vi "xml_lib Implementation.vi"(8 "error in (no error)":errorcluster, 11 "class path":path) -> (0 "error out":errorcluster, 3 "Array":path[](array[path]))   [LabVIEW 2020, in "Test Method Finding Test.lvclass"]
uses:
  Test Method Finding Test.lvclass
  <vilib>/xml/Load XML File.vi
  <vilib>/xml/Close Reference(Node).vi
  Test Method Finding Test.lvclass/Test Method Finding Test.ctl
  <resource>/objmgr/DOMUserDefRef.rc
  <vilib>/xml/NI_XML.lvlib
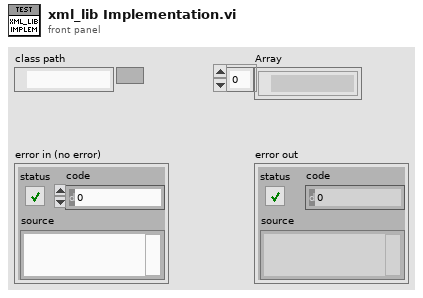
[diagram p1: front panel]
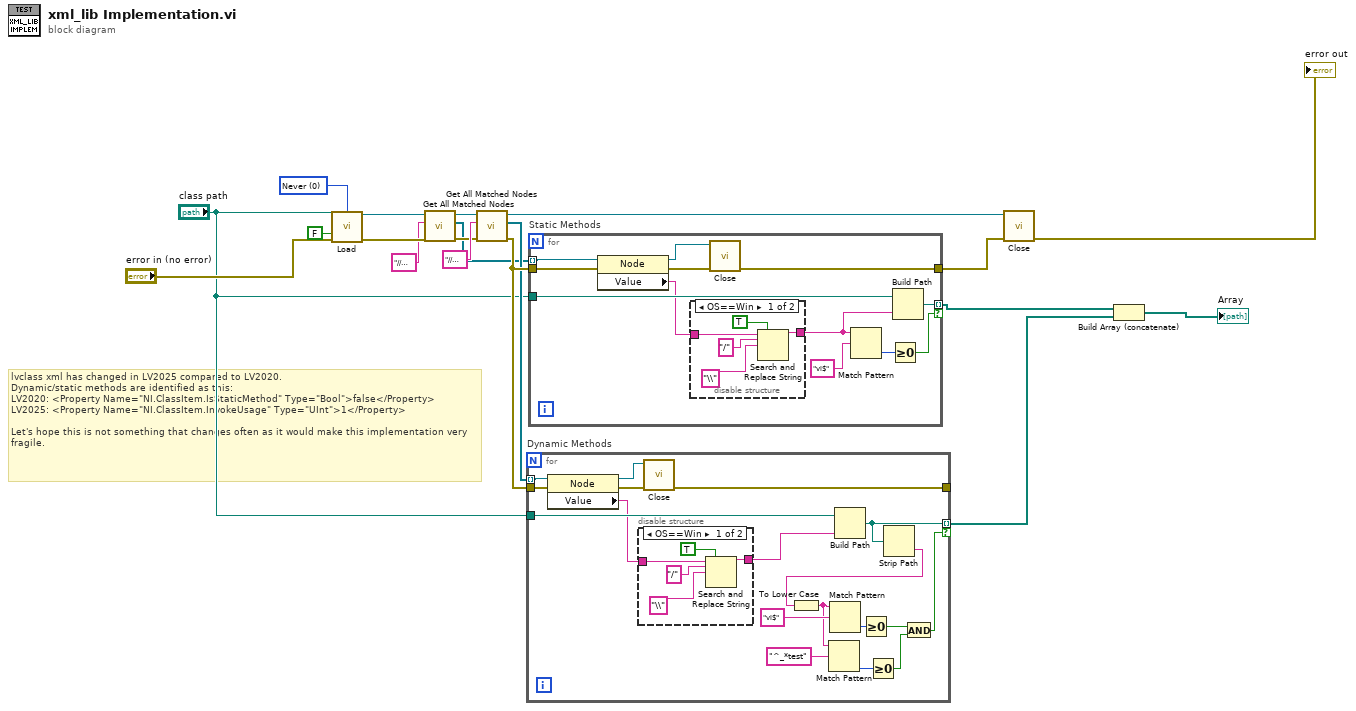
[diagram p0: block diagram]
diagram:
  w5 = 0 items=["Never", "Always", "Auto"] ("validate on load (Auto)")
  # "lvclass xml has changed in LV2025 compared to LV2020.\nDynamic/static methods are identified as this:\nLV2020: <Property Name=\"NI.ClassItem.IsStaticMethod\" Type=\"Bool\">false</Property>\nLV2025: <Property Name=\"NI.ClassItem.InvokeUsage\" Type=\"UInt\">1</Property>\n\nLet's hope this is not something that changes often as it would make this implementation very fragile."
  n1 = call-poly <vilib>:"Load.vi"("path to XML document"="class path", "validate on load (Auto)"=w5, "load external DTD (True)"=FALSE, "error in (no error)"="error in (no error)") -> ("DOM document out"=w7:refnum<k20>, "error out"=w11:errorcluster)  [unwired: 9 in, 1 out]
  n2 = call <vilib>:"Get All Matched Nodes.vi"("error in (no error)"=w11, "XPath expression"="//Item[@Type='VI'][Property[@Name='NI.ClassItem.InvokeUsage']='0'\n    or Property[@Name='NI.ClassItem.IsStaticMethod']='true'][Property[@Name='NI.ClassItem.MethodScope']='1']/@URL", "node in"=w7) -> ("error out"=w14:errorcluster, "node result array"=w9:refnum<k20>[], "node out"=w12:refnum<k20>)  [unwired: 6 out]
  n3 = call <vilib>:"Get All Matched Nodes.vi"("error in (no error)"=w14, "XPath expression"="//Item[@Type='VI'][Property[@Name='NI.ClassItem.InvokeUsage']='1'\n    or Property[@Name='NI.ClassItem.IsStaticMethod']='false'][Property[@Name='NI.ClassItem.MethodScope']='1']/@URL", "node in"=w12) -> ("error out"=w17:errorcluster, "node result array"=w16:refnum<k20>[], "node out"=w13:refnum<k20>)  [unwired: 6 out]
  n4 = for "Dynamic Methods" {
    tunnel: w16 -> [w37] mode=indexing
    tunnel: w17 -> [w36]
    tunnel: [w33] -> _
    tunnel: "class path" -> [w32]
    tunnel: [w24] -> w4 mode=indexing if=w25
    n5 = property class="Node"(reference=w37, error in=w36) -> (reference out=w35:refnum<k20>, error out=w34:errorcluster, "Value"=w21:string)
    n6 = disable-structure shown="OS==Win" {
      disable-tunnel: [w41 w43] -> w20
      disable-tunnel: w21 -> [w40 w43]
      frame condition #0 (active) {
        n7 = Search and Replace String(replace all?=TRUE ("replace all? (F)"), input string=w40, search string="/", replace string="\\" ("search string")) -> (result string=w41:string)  [unwired: 4 in, 3 out]
      }
      frame condition #1 {
      }
    }
    n8 = call-poly <vilib>:"Close.vi"("error in (no error)"=w34, "node"=w35) -> ("error out"=w33:errorcluster)  [unwired: 7 out]
    n9 = Build Path(base path=w32, name or relative path=w20) -> (appended path=w24:path)
    n10 = Strip Path(path=w24) -> (name=w23:string)  [unwired: 1 out]
    n11 = To Lower Case(string=w23) -> (all lower case string=w22:string)
    n12 = Match Pattern(string=w22, regular expression="^_*test") -> (offset past match=w29:i32)  [unwired: 1 in, 3 out]
    n13 = Match Pattern(string=w22, regular expression="vi$") -> (offset past match=w30:i32)  [unwired: 1 in, 3 out]
    n14 = Greater Or Equal To 0?(x=w30) -> (x >= 0?=w26:bool)
    n15 = Greater Or Equal To 0?(x=w29) -> (x >= 0?=w27:bool)
    n16 = And(x=w26, y=w27) -> (x .and. y?=w25:bool)
  }
  n17 = for "Static Methods" {
    tunnel: w9 -> [w55] mode=indexing
    tunnel: w17 -> [w54]
    tunnel: [w51] -> w10
    tunnel: "class path" -> [w50]
    tunnel: [w49] -> w2 mode=indexing if=w45
    n18 = property class="Node"(reference=w55, error in=w54) -> (reference out=w53:refnum<k20>, error out=w52:errorcluster, "Value"=w48:string)
    n19 = disable-structure shown="OS==Win" {
      disable-tunnel: [w59 w61] -> w44
      disable-tunnel: w48 -> [w58 w61]
      frame condition #0 (active) {
        n20 = Search and Replace String(replace all?=TRUE ("replace all? (F)"), input string=w58, search string="/", replace string="\\" ("search string")) -> (result string=w59:string)  [unwired: 4 in, 3 out]
      }
      frame condition #1 {
      }
    }
    n21 = call-poly <vilib>:"Close.vi"("error in (no error)"=w52, "node"=w53) -> ("error out"=w51:errorcluster)  [unwired: 7 out]
    n22 = Match Pattern(string=w44, regular expression="vi$") -> (offset past match=w46:i32)  [unwired: 1 in, 3 out]
    n23 = Greater Or Equal To 0?(x=w46) -> (x >= 0?=w45:bool)
    n24 = Build Path(base path=w50, name or relative path=w44) -> (appended path=w49:path)
  }
  n25 = call-poly <vilib>:"Close.vi"("error in (no error)"=w10, "node"=w13) -> ("error out"=→"error out":errorcluster)  [unwired: 7 out]
  n26 = Build Array (concatenate)(w2, w4) -> (→"Array":path[])
